vi "Init Hardware.vi"(8 "error in (no error)":errorcluster, 11 "HP Counter Driver in":refnum<class "HP Counter Driver.lvclass">) -> (0 "error out":errorcluster, 3 "HP Counter Driver out":refnum<class "HP Counter Driver.lvclass">)   [LabVIEW 2016, in "HP Counter Driver.lvclass"]
uses:
  HP Counter Driver.lvclass
  C:/github/NHMFL_Core/Libraries/Instruments/Instrument Driver/Instrument Driver.lvclass
  Instrument Driver/Instrument Driver.lvclass/Instrument Driver.ctl
  Instrument Driver/Read Recorder name.vi
  Instrument Driver/Write Channel names.vi
  Instrument Driver/Write Channel units.vi
  Simple VISA Reader/Simple VISA Reader Driver.lvclass
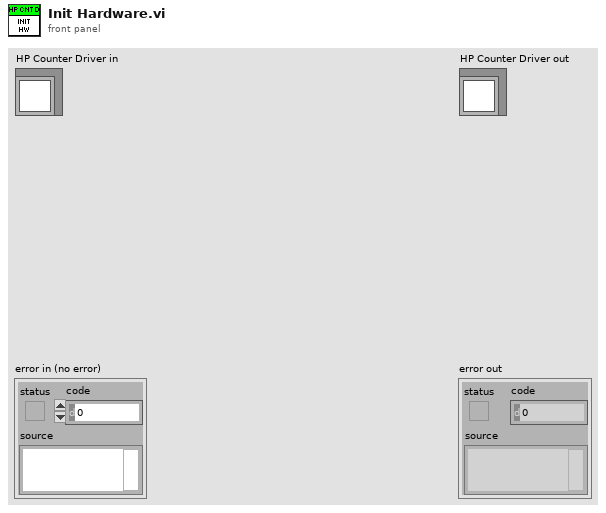
[diagram p1: front panel]
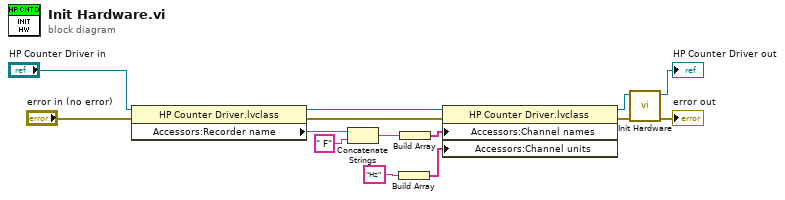
[diagram p0: block diagram]
diagram:
  n1 = property class="HP Counter Driver.lvclass"(reference="HP Counter Driver in", error in="error in (no error)") -> (reference out=w6:refnum<class "HP Counter Driver.lvclass">, error out=w5:errorcluster, "Accessors:Recorder name"=w11:string)
  n2 = Concatenate Strings(w11, " F") -> (w10:string)
  n3 = Build Array("Hz") -> (w7:string[])
  n4 = Build Array(w10) -> (w8:string[])
  n5 = property class="HP Counter Driver.lvclass"(reference=w6, error in=w5, "Accessors:Channel names"=w8, "Accessors:Channel units"=w7) -> (reference out=w3:refnum<class "HP Counter Driver.lvclass">, error out=w2:errorcluster)
  n6 = call-parent "Init Hardware.vi"("error in (no error)"=w2, "Instrument Driver in"=w3) -> ("error out"=→"error out":errorcluster, "Instrument Driver out"=→"HP Counter Driver out":refnum<class "HP Counter Driver.lvclass">)  [unwired: 8 in]
